vi "sender_daq.vi"(10 "address":string) -> ()   [LabVIEW 2013]
panel:
  in  "Boolean":bool
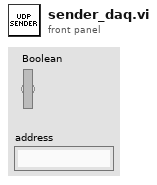
[diagram p1: front panel]
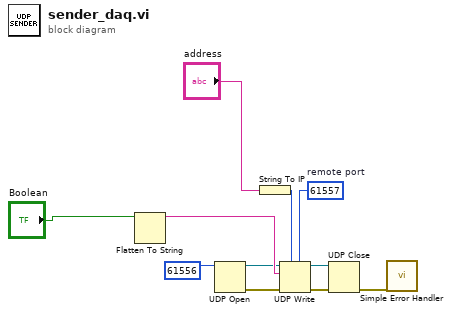
[diagram p0: block diagram]
diagram:
  w5 = u16 61557  # remote port
  n1 = Flatten To String(anything="Boolean") -> (data string=w11:string)  [unwired: 3 in, 2 out]
  n2 = UDP Open(11:u16 61556) -> (port=w7:refnum<k16>, 0:w8:errorcluster)  [unwired: 4 in, 1 out]
  n3 = String To IP(1:"address") -> (0:w6:u32)
  n4 = UDP Write(address=w6, port or service name=w5, connection ID=w7, data in=w11, 8:w8) -> (error out=w10:errorcluster, 3:w9:refnum<k16>)  [unwired: 1 in]
  n5 = UDP Close(connection ID=w9, 8:w10) -> (error out=w3:errorcluster)  [unwired: 1 out]
  n6 = call <vilib>:"Simple Error Handler.vi"("error in (no error)"=w3) -> ()  [unwired: 4 in, 5 out]
